vi "Keep Alive.vi"(8 "error in (no error)":errorcluster, 9 "Connection Name":string) -> (0 "error out":errorcluster)   [LabVIEW 2017, in "LabSFTP.lvlib"]
doc: "<License>This software is distributed under the BSD 3-Clause License. For the full license please see license.txt or visit www.labvolution.com/license</License>"
uses:
  LabSFTP.lvlib
  FGV State..enum.ctl
  C:/Users/OCT/Downloads/LabSSH-Library-2015/LabSSH Library/References/LabSFTP.dll
  Downloads/LabSSH-Library-2015/LabSSH Library/References/LabSFTP.dll
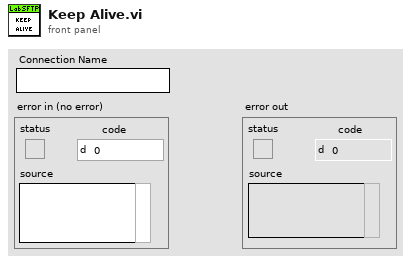
[diagram p1: front panel]
types:
  T1 = typedef "LabSFTP.lvlib/FGV State..enum.ctl" = enum16{"GET", "SET"}
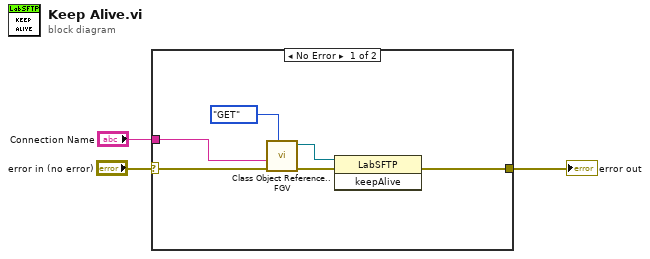
[diagram p0: block diagram]
diagram:
  n1 = case shown="No Error" "error in (no error)" {
    selector: "error in (no error)" -> [w6 w10]
    tunnel: [w5 w10] -> w2
    tunnel: "Connection Name" -> [w4 _]
    frame No Error {
      n2 = call "Class Object Reference..FGV.vi"("FGV State"=FGV_State..enum."GET", "error in (no error)"=w6, "Connection Name"=w4) -> ("error out"=w7:errorcluster, "LabSFTP ref out"=w8:refnum<k24>)  [unwired: 7 in]
      n3 = invoke on="Invoke Node" class="LabSFTP" method="keepAlive"(reference=w8, error in=w7) -> (error out=w5:errorcluster)  [unwired: 1 in, 2 out]
    }
    frame Error {
    }
  }
  "error out" <- w2
